vi "readSGLFIFO.vi"(8 "error in (no error)":errorcluster, 9 "Timeout":i32, 10 "NumberOfElements":u32, 11 "MyHealthAndStatusReadFIFO in":refnum<class "Accel1Channel1FIFO.lvclass">) -> (0 "error out":errorcluster, 1 "ElementsRemaining":u32, 2 "Data":sgl[](array[numeric]), 3 "MyHealthAndStatusReadFIFO out":refnum<class "Accel1Channel1FIFO.lvclass">)   [LabVIEW 2016, in "Accel1Channel1FIFO.lvclass"]
uses:
  Accel1Channel1FIFO.lvclass
  Accel1Channel1FIFO.lvclass/Accel1Channel1FIFO.ctl
  <vilib>/Utility/error.llb/Error Cluster From Error Code.vi
  <vilib>/rvi/errors/niLvFpgaAdjustHostInterfaceError.vi
  <vilib>/rvi/interface/nirviMethod/nirviMethod.xnode
  <vilib>/FPGAPlugInAG/Dynamic/niLvFpga_ReadFifo_Dynamic.vi
  <vilib>/rvi/errors/niLvFpgaMergeErrorWithErrorCode.vi
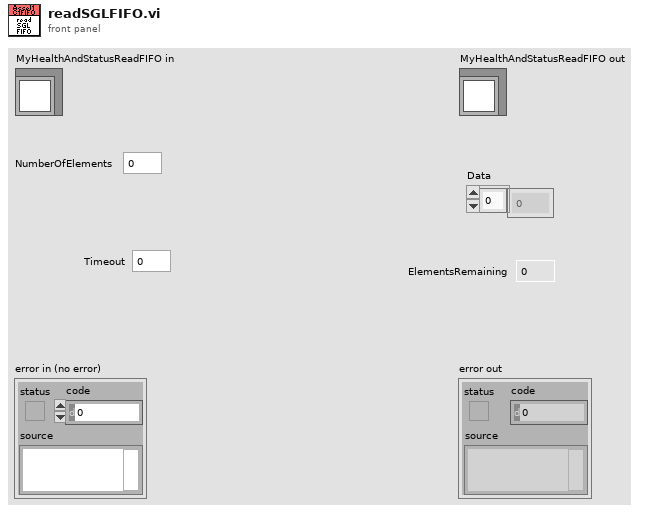
[diagram p1: front panel]
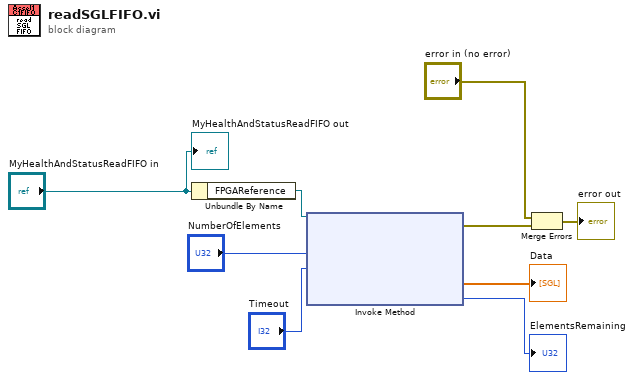
[diagram p0: block diagram]
diagram:
  n1 = Unbundle By Name("MyHealthAndStatusReadFIFO in") -> ("FPGAReference"=w9:refnum<k20>)
  n2 = xnode "Invoke Method"("FPGA VI Reference In"=w9, "Number of Elements"="NumberOfElements", "Timeout (ms)"="Timeout") -> ("error out"=w2:errorcluster, "Data"=→"Data":sgl[], "Elements Remaining"=→"ElementsRemaining":u32)  [unwired: 1 in, 1 out]
  n3 = Merge Errors("error in (no error)", w2) -> (→"error out":errorcluster)
  "MyHealthAndStatusReadFIFO out" <- "MyHealthAndStatusReadFIFO in"
